vi "Write VacuumLine Obj.vi"(8 "error in (no error)":errorcluster, 10 "Hardware.lvlib:VacuumLine.lvlib:VacuumLine.lvclass":refnum<class "VacuumLine.lvclass">, 11 "VacuumLine Configuration in":refnum<class "VacuumLine Configuration.lvclass">) -> (0 "error out":errorcluster, 3 "VacuumLine Configuration out":refnum<class "VacuumLine Configuration.lvclass">)   [LabVIEW 2016, in "Hardware.lvlib" / "VacuumLine.lvlib" / "VacuumLine Configuration.lvclass"]
uses:
  <userlib>/Common Components/Hardware/Abstract System/VacuumLine/VacuumLine Config/VacuumLine Configuration.lvclass
  <userlib>/Common Components/Hardware/Abstract System/VacuumLine/VacuumLine/VacuumLine.lvclass
  <userlib>/Common Components/Hardware/Abstract System/VacuumLine/VacuumLine Config/VacuumLine Configuration.lvclass/VacuumLine Configuration.ctl
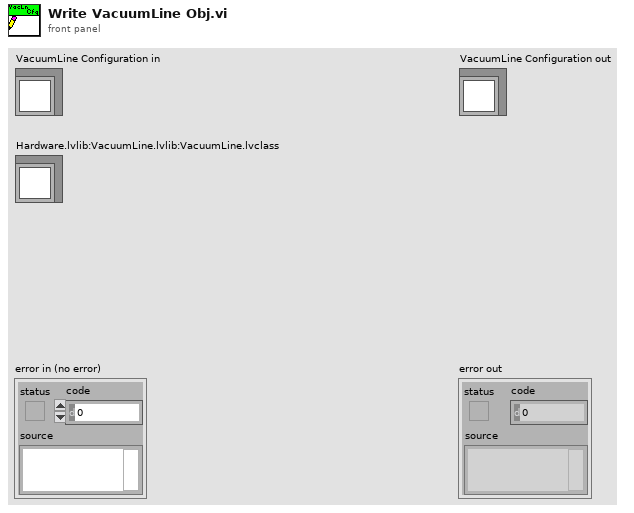
[diagram p1: front panel]
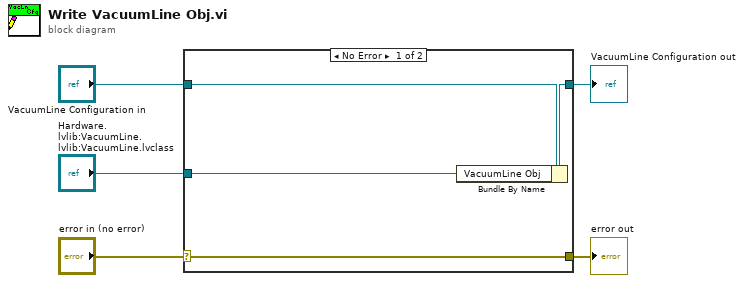
[diagram p0: block diagram]
diagram:
  n1 = case shown="No Error" "error in (no error)" {
    selector: "error in (no error)" -> [w9 w10]
    tunnel: [w9 w10] -> w4
    tunnel: [w7 w11] -> w2
    tunnel: "VacuumLine Configuration in" -> [w8 w11]
    tunnel: "Hardware.lvlib:VacuumLine.lvlib:VacuumLine.lvclass" -> [w6 _]
    frame No Error {
      n2 = Bundle By Name(cluster=w8, "VacuumLine Obj"=w6) -> (w7:refnum<class "VacuumLine Configuration.lvclass">)
    }
    frame Error {
    }
  }
  "error out" <- w4
  "VacuumLine Configuration out" <- w2
